vi "thermometer1.vi"(8 "error in (no error)":errorcluster, 11 "module name":string="thermometer1") -> (0 "error out":errorcluster)   [LabVIEW 2019]
doc: "The specification of a thermometer is to report the temperature every tick to the topic \"env\". For logging, report messages to \"log\". All data in and out is type String.\n\nWhen this version of the thermometer is initialized, the thermometer will report in Celsius and every 20 ms.\n\nOptions:\nThis module should listen to msg \"unit\" with data \"C\", \"F\", or \"K\" to convert the units to C, F, or K, respectively.\nThis module should listen to msg \"rate\" to change the update rate; valid values are betwen 1 and 100 ms.\nIf invalid values are provided, ignore the value but report it to \"log\"."
uses:
  common/common data types/common_event_data.ctl
panel:
  out "sampling period [ms]":string
  out "units":string
  out "temperature reported":dbl(slide) scale=0.0..350.0
  out "new temperature in C":dbl(slide) scale=0.0..100.0
  out "global stop?":bool
  in  "stop this module":bool
  out "targetted":bool
  out "target":string
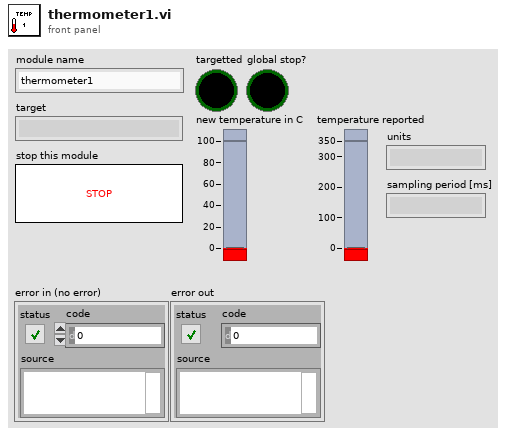
[diagram p1: front panel]
types:
  T1 = typedef "common_event_data.ctl" = cluster{"sender":string, "target":string, "msg":string, "data":variant}
  T2 = cluster{"module name":string, "units (C)":string, "period (20)":string}
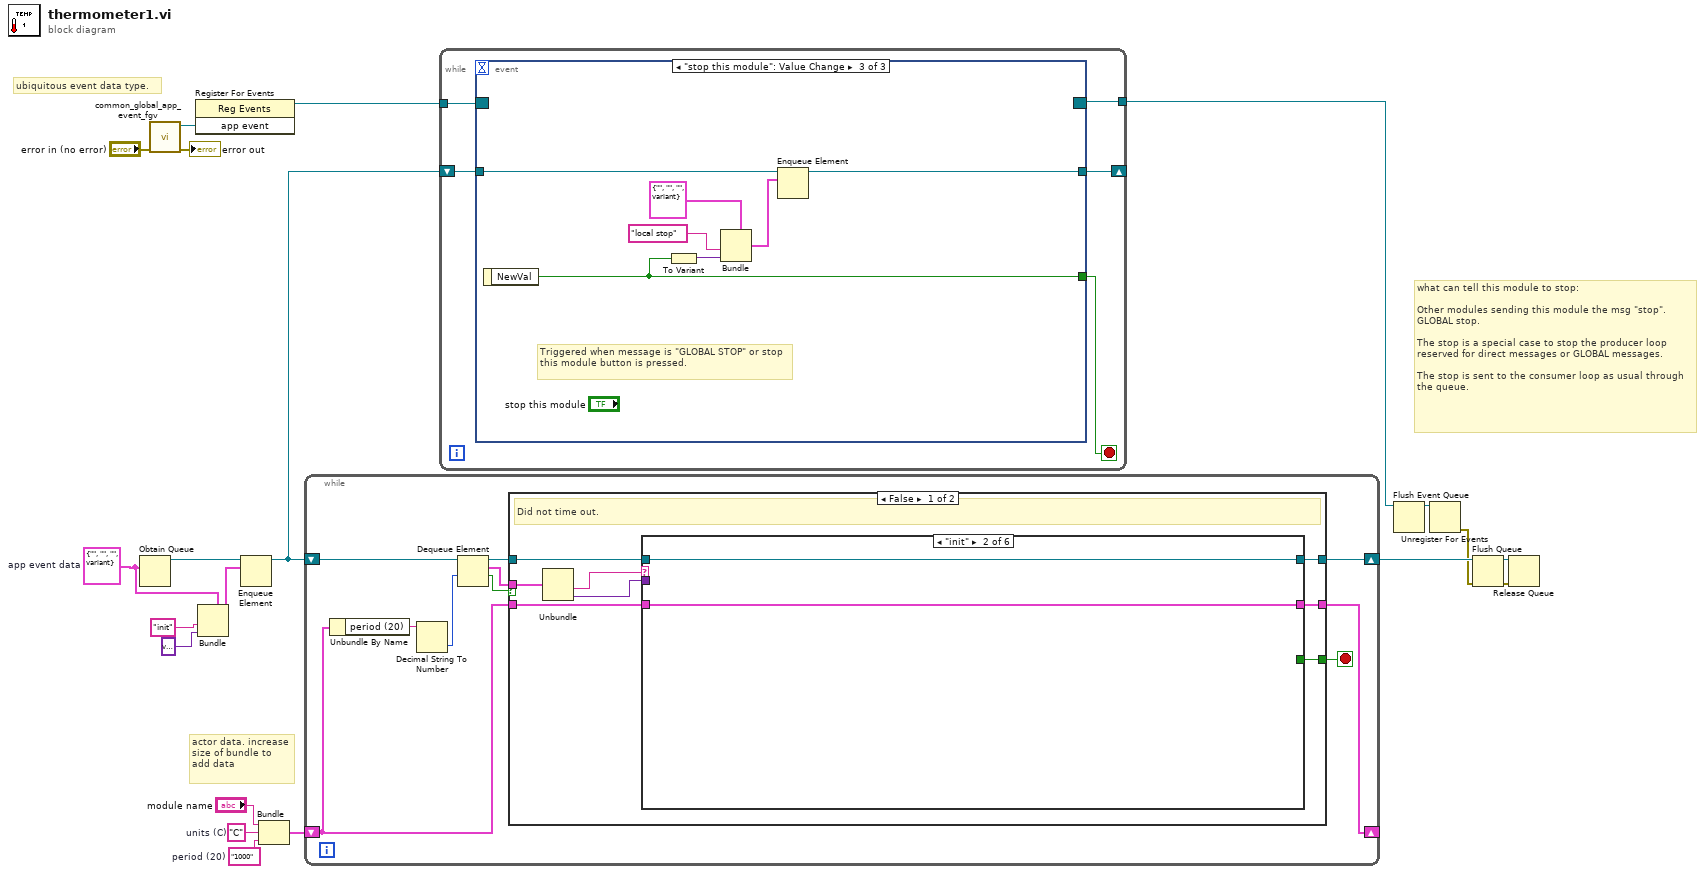
[diagram p0: block diagram]
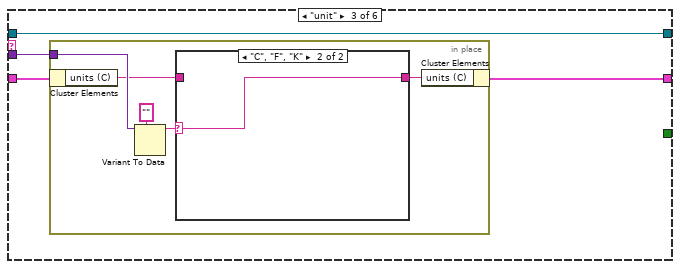
[diagram p3: hidden frame]
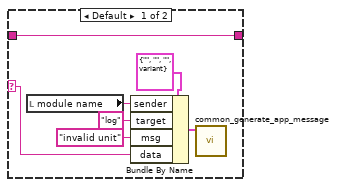
[diagram p4: hidden frame]
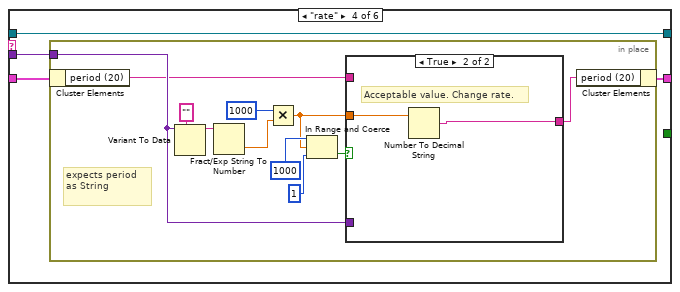
[diagram p5: hidden frame]
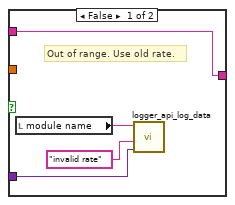
[diagram p6: hidden frame]
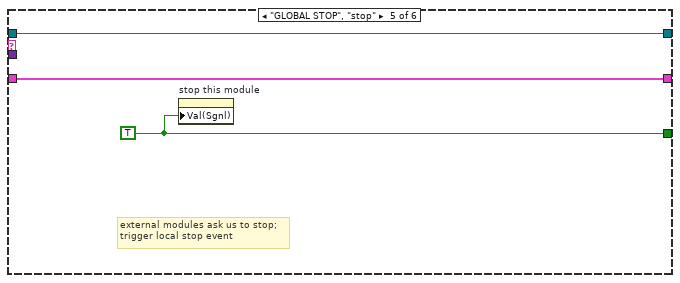
[diagram p7: hidden frame]
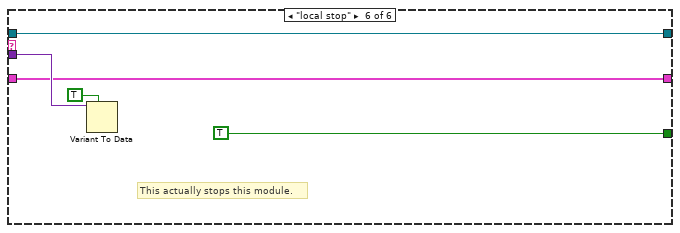
[diagram p8: hidden frame]
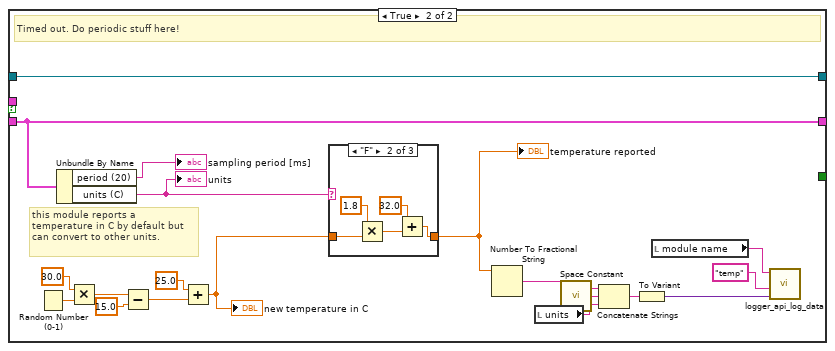
[diagram p9: hidden frame]
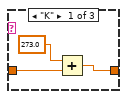
[diagram p10: hidden frame]
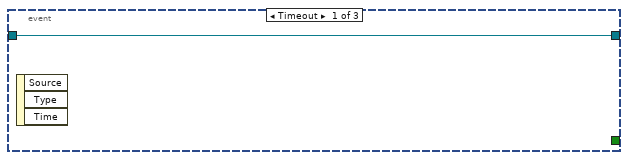
[diagram p12: hidden frame]
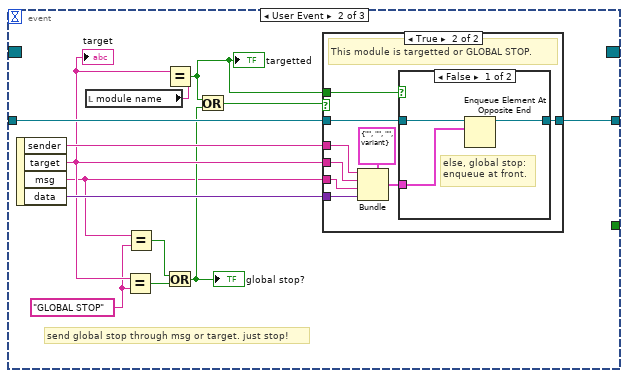
[diagram p13: hidden frame]
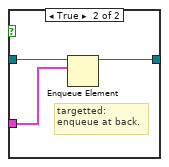
[diagram p15: hidden frame]
diagram:
  w3 = "1000"  # period (20)
  w5 = "C"  # units (C)
  w9 = T1 {"sender"="", "target"="", "msg"="", "data"=variant}  # app event data
  # "actor data. increase size of bundle to add data"
  # "what can tell this module to stop:\n\nOther modules sending this module the msg \"stop\".\nGLOBAL stop.\n\nThe stop is a special case to stop the producer loop reserved for direct messages or GLOBAL messages.\n\nThe stop is sent to the consumer loop as usual through the queue."
  # "ubiquitous event data type."
  n1 = Obtain Queue(element data type=w9) -> (queue out=w20:refnum<queue>)  [unwired: 4 in, 2 out]
  n2 = call "common_global_app_event_fgv.vi"("error in (no error)"="error in (no error)") -> ("error out"=→"error out":errorcluster, "app event"=w14:refnum<user-event>)  [unwired: 9 in]
  n3 = register-events(w14) -> (reference out=w15:refnum<event-registration>)  [unwired: 2 in, 1 out]
  n4 = Bundle(cluster=w9, "msg"="init" ("target"), "data"=variant) -> (w19:T1)  [unwired: 2 in]
  n5 = Enqueue Element(queue=w20, element=w19) -> (queue out=w18:refnum<queue>)  [unwired: 2 in, 2 out]
  n6 = Bundle("module name"="module name", "units (C)"=w5, "period (20)"=w3) -> (w6:T2)  [unwired: 1 in]
  n7 = while {
    shift-right: [w27] -> w16
    shift-left: w18 -> [w30]
    shift-right: [w24] -> _
    shift-left: w6 -> [w23]
    stop <- w26 stop-if-true
    n8 = Unbundle By Name(w23) -> ("period (20)"=w21:string)
    n9 = Decimal String To Number(string=w21) -> (number=w22:i32)  [unwired: 2 in, 1 out]
    n10 = Dequeue Element(queue=w30, timeout in ms (-1)=w22) -> (queue out=w28:refnum<queue>, element=w29:T1, timed out?=w25:bool)  [unwired: 1 in, 1 out]
    n11 = case shown="False" w25 {
      tunnel: w29 -> [w38 _]
      tunnel: w28 -> [w37 w107]
      tunnel: [w36 w107] -> w27
      tunnel: [w35 _] -> w26
      tunnel: w23 -> [w32 w100]
      tunnel: [w31 w100] -> w24
      frame False {
        # "Did not time out."
        n12 = Unbundle(w38) -> ("msg"=w33:string, "data"=w34:variant)  [unwired: 2 out]
        n13 = case shown="\"init\"" w33 {
          tunnel: w37 -> [w40 w42 w45 w62 w83 w88]
          tunnel: [w40 w42 w45 w62 w83 w88] -> w36
          tunnel: w34 -> [_ _ w44 w61 _ w86]
          tunnel: [_ _ _ _ w82 TRUE] -> w35
          tunnel: w32 -> [w39 w41 w46 w63 w81 w84]
          tunnel: [w39 w41 w43 w60 w81 w84] -> w31
          frame Default {
            # "unsupported message."
          }
          frame "init" {
          }
          frame "unit" {
            n14 = in-place {
              in-place-border: w44 -> [w51]
              n15 = in-place-cluster #1(w46) -> ("units (C)"=w47:string)
              n16 = Variant To Data(type="", Variant=w51) -> (data=w49:string)  [unwired: 1 in, 1 out]
              n17 = case shown="\"C\", \"F\", \"K\"" w49 {
                selector: w49 -> [w52 w59]
                tunnel: [w58 w59] -> w48
                tunnel: w47 -> [w58 _]
                frame Default {
                  n18 = local read "module name"() -> (w57:string)
                  n19 = Bundle By Name(cluster=T1 {"sender"="", "target"="", "msg"="", "data"=variant} ("event data"), "sender"=w57, "target"="log", "msg"="invalid unit", "data"=w52) -> (w56:T1)
                  n20 = call "common_generate_app_message.vi"("event data"=w56) -> ()  [unwired: 10 in, 1 out]
                }
                frame "C", "F", "K" {
                }
              }
              n21 = in-place-cluster #1("units (C)"=w48) -> (w43:T2)
            }
          }
          frame "rate" {
            n22 = in-place {
              in-place-border: w61 -> [w70]
              # "expects period as String"
              n23 = in-place-cluster #2(w63) -> ("period (20)"=w68:string)
              n24 = Variant To Data(type="", Variant=w70) -> (data=w71:string)  [unwired: 1 in, 1 out]
              n25 = Fract/Exp String To Number(string=w71) -> (number=w66:dbl)  [unwired: 3 in, 1 out]
              n26 = Multiply(x=1000, y=w66) -> (x*y=w64:dbl)
              n27 = In Range and Coerce(upper limit=1000 ("default (0 I32)"), x=w64, lower limit=1 ("default (0 I32)")) -> (In Range?=w72:bool)  [unwired: 1 out]
              n28 = case shown="True" w72 {
                tunnel: [w78 w79] -> w69
                tunnel: w70 -> [w75 _]
                tunnel: w68 -> [w78 _]
                tunnel: w64 -> [_ w80]
                frame False {
                  # "Out of range. Use old rate."
                  n29 = local read "module name"() -> (w77:string)
                  n30 = call "logger_api_log_data.vi"("data"=w75, "msg"="invalid rate", "sender"=w77) -> ()  [unwired: 9 in]
                }
                frame True {
                  # "Acceptable value. Change rate."
                  n31 = Number To Decimal String(number=w80) -> (decimal integer string=w79:string)  [unwired: 1 in]
                }
              }
              n32 = in-place-cluster #2("period (20)"=w69) -> (w60:T2)
            }
          }
          frame "GLOBAL STOP", "stop" {
            w82 = TRUE
            # "external modules ask us to stop;\ntrigger local stop event"
            n33 = property on="stop this module" class="Bool (strict)"("Val(Sgnl)"=w82) -> ()  [unwired: 2 in, 2 out]
          }
          frame "local stop" {
            # "This actually stops this module."
            n34 = Variant To Data(type=TRUE, Variant=w86) -> ()  [unwired: 1 in, 2 out]
          }
        }
      }
      frame True {
        # "this module reports a temperature in C by default but can convert to other units."
        # "Timed out. Do periodic stuff here!"
        n35 = Random Number (0-1)() -> (number: 0 to 1=w104:dbl)
        n36 = Unbundle By Name(w100) -> ("period (20)"=→"sampling period [ms]":string, "units (C)"=w99:string)
        "units" <- w99
        n37 = Multiply(x=30.0, y=w104) -> (x*y=w105:dbl)
        n38 = Subtract(x=w105, y=15.0) -> (x-y=w106:dbl)
        n39 = Add(x=25.0, y=w106) -> (x+y=w98:dbl)
        "new temperature in C" <- w98
        n40 = case shown="\"F\"" w99 {
          tunnel: w98 -> [w110 w113 w116]
          tunnel: [w109 w111 w116] -> w97
          frame "K" {
            n41 = Add(x=273.0, y=w110) -> (x+y=w109:dbl)
          }
          frame "F" {
            n42 = Multiply(x=1.8, y=w113) -> (x*y=w115:dbl)
            n43 = Add(x=32.0, y=w115) -> (x+y=w111:dbl)
          }
          frame "C", Default {
          }
        }
        "temperature reported" <- w97
        n44 = Number To Fractional String(number=w97) -> (F-format string=w90:string)  [unwired: 3 in]
        n45 = local read "units"() -> (w91:string)
        n46 = call <vilib>:"Space Constant.vi"() -> ("String"=w92:string)
        n47 = Concatenate Strings(w90, w92, w91) -> (w89:string)
        n48 = To Variant(anything=w89) -> (Variant=w94:variant)
        n49 = local read "module name"() -> (w96:string)
        n50 = call "logger_api_log_data.vi"("data"=w94, "msg"="temp", "sender"=w96) -> ()  [unwired: 9 in]
      }
    }
  }
  n51 = while {
    tunnel: w15 -> [w121]
    shift-right: [w119] -> _
    shift-left: w18 -> [w120]
    tunnel: [w118] -> w2
    stop <- w117 stop-if-true
    n52 = event shown="[2] \"stop this module\": Value Change" {
      selector: w121 -> [_ _ _]
      dyn-events: [_ _ _] -> w118
      timeout: _ -> [_ _ _]
      tunnel: w120 -> [w122 w134 w156]
      tunnel: [w122 w133 w157] -> w119
      tunnel: [_ _ w152] -> w117
      event Timeout {
        n53 = event-data() -> ()  [unwired: 1 in, 3 out]
      }
      event User Event {
        w126 = "GLOBAL STOP"
        # "send global stop through msg or target. just stop!"
        n54 = event-data() -> ("sender"=w132:string, "target"=w131:string, "msg"=w125:string, "data"=w135:variant)  [unwired: 1 in]
        "target" <- w131
        n55 = local read "module name"() -> (w123:string)
        n56 = Equal?(x=w131, y=w126) -> (x = y?=w128:bool)
        n57 = Equal?(x=w125, y=w126) -> (x = y?=w124:bool)
        n58 = Equal?(x=w131, y=w123) -> (x = y?=w129:bool)
        "targetted" <- w129
        n59 = Or(x=w124, y=w128) -> (x .or. y?=w127:bool)
        "global stop?" <- w127
        n60 = Or(x=w129, y=w127) -> (x .or. y?=w130:bool)
        n61 = case shown="True" w130 {
          tunnel: w125 -> [_ w141]
          tunnel: w135 -> [_ w142]
          tunnel: w134 -> [w136 w145]
          tunnel: [w136 w144] -> w133
          tunnel: w131 -> [_ w140]
          tunnel: w132 -> [_ w139]
          tunnel: w129 -> [_ w137]
          frame False {
          }
          frame True {
            # "This module is targetted or GLOBAL STOP."
            n62 = Bundle(cluster=T1 {"sender"="", "target"="", "msg"="", "data"=variant}, "sender"=w139, "target"=w140, "msg"=w141, "data"=w142) -> (w138:T1)
            n63 = case shown="False" w137 {
              tunnel: w145 -> [w148 w151]
              tunnel: [w147 w150] -> w144
              tunnel: w138 -> [w146 w149]
              frame False {
                # "else, global stop: \nenqueue at front."
                n64 = Enqueue Element At Opposite End(queue=w148, element=w146) -> (queue out=w147:refnum<queue>)  [unwired: 2 in, 2 out]
              }
              frame True {
                # "targetted:\nenqueue at back."
                n65 = Enqueue Element(queue=w151, element=w149) -> (queue out=w150:refnum<queue>)  [unwired: 2 in, 2 out]
              }
            }
          }
        }
      }
      event "stop this module": Value Change {
        # "Triggered when message is \"GLOBAL STOP\" or stop this module button is pressed."
        n66 = event-data() -> ("NewVal"=w152:bool)  [unwired: 1 in]
        n67 = To Variant(anything=w152) -> (Variant=w153:variant)
        n68 = Bundle(cluster=T1 {"sender"="", "target"="", "msg"="", "data"=variant}, "msg"="local stop", "data"=w153) -> (w158:T1)  [unwired: 2 in]
        n69 = Enqueue Element(queue=w156, element=w158) -> (queue out=w157:refnum<queue>)  [unwired: 2 in, 2 out]
      }
    }
  }
  n70 = Flush Event Queue(0:w2) -> (8:w1:refnum<event-registration>)  [unwired: 5 in, 2 out]
  n71 = Unregister For Events(event registration refnum=w1) -> (error out=w11:errorcluster)  [unwired: 1 in]
  n72 = Flush Queue(queue=w16, error in (no error)=w11) -> (queue out=w17:refnum<queue>, error out=w10:errorcluster)  [unwired: 1 out]
  n73 = Release Queue(queue=w17, error in (no error)=w10) -> ()  [unwired: 1 in, 3 out]
